vi "Open.vi"(8 "error in (no error)":errorcluster, 11 "Enabled Frames":T2={"Color"=TRUE, "Infrared"=TRUE, "LongExposureInfrared"=TRUE, "Depth"=TRUE, "BodyIndex"=TRUE, "Body"=TRUE}) -> (0 "error out":errorcluster, 3 "KinectSensor References out":T1)   [LabVIEW 2014, in "LVH-KinectOne.lvlib"]
uses:
  LVH-KinectOne.lvlib
  Private/Type Defs/KinectSensor References.ctl
  Microsoft.Kinect
  C:/github/labviewhacker/LVH-KinectOne/LabVIEW/vi.lib/LabVIEW Hacker/KinectOne/Private/Libs/BodyFrameDataInterface.dll
  Private/Libs/BodyFrameDataInterface.dll
  Private/Type Defs/FrameDescription.ctl
  Private/Frame Description FGV [Color].vi
  Private/Frame Data FGV [Color].vi
  Private/Frame Description FGV [Infrared].vi
  Private/Frame Data FGV [Infrared].vi
  Private/Frame Description FGV [Long Exposure Infrared].vi
  Private/Frame Data FGV [Long Exposure Infrared].vi
  Private/Frame Description FGV [Depth].vi
  Private/Frame Data FGV [Depth].vi
  Private/Frame Description FGV [Body Index].vi
  Private/Frame Data FGV [Body Index].vi
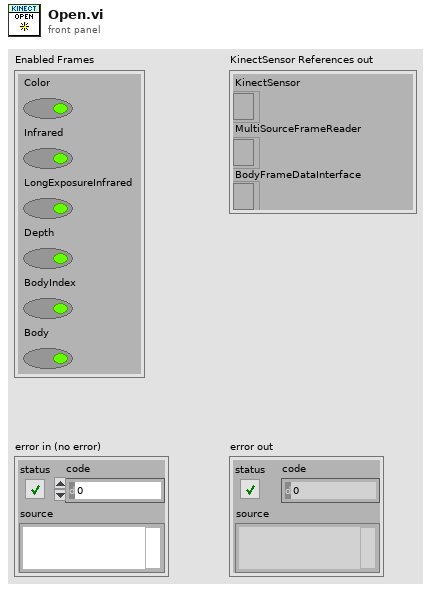
[diagram p1: front panel]
types:
  T1 = typedef "LVH-KinectOne.lvlib/KinectSensor References.ctl" = cluster{"KinectSensor":refnum<k24>, "MultiSourceFrameReader":refnum<k24>, "BodyFrameDataInterface":refnum<k24>}
  T2 = cluster{"Color":bool, "Infrared":bool, "LongExposureInfrared":bool, "Depth":bool, "BodyIndex":bool, "Body":bool}
  T3 = typedef "LVH-KinectOne.lvlib/FrameDescription.ctl" = cluster{"BytesPerPixel":u32, "DiagonalFieldOfView":sgl, "Height":i32, "HorizontalFieldOfView":sgl, "LengthInPixels":u32, "VerticalFieldOfView":sgl, "Width":i32}
  T4 = enum16{"Get Joint Position", "Initialize", "Set Joint Position"}
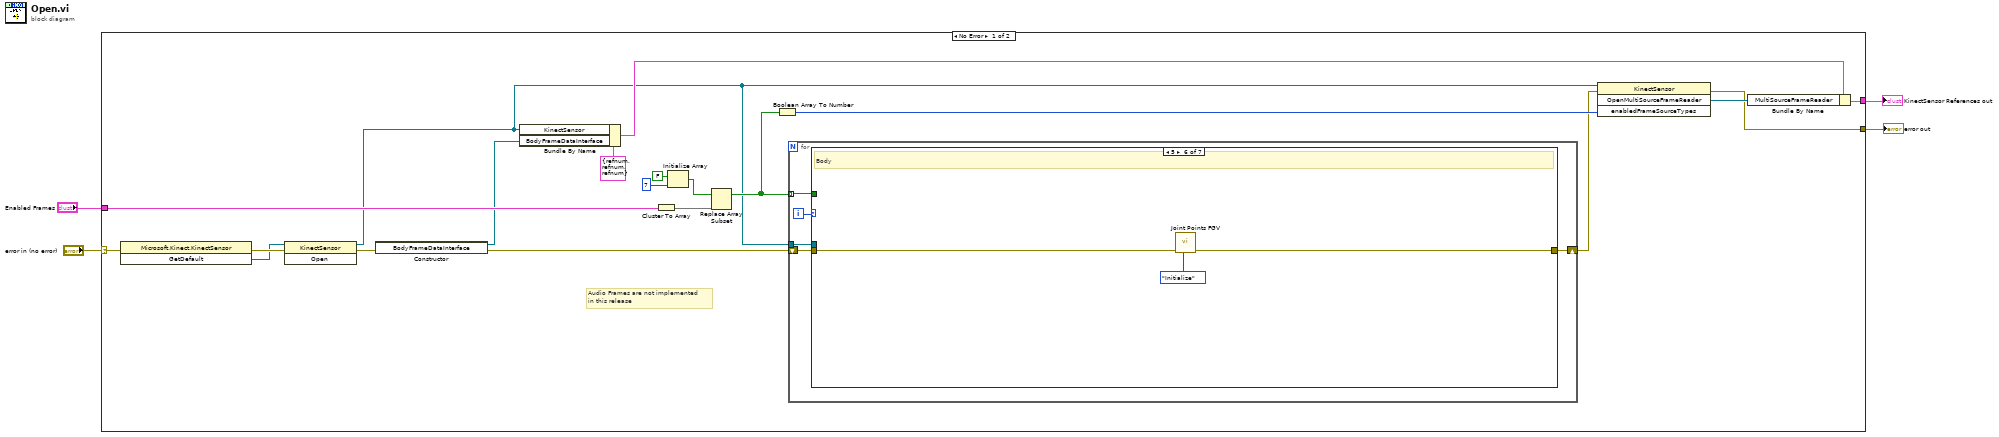
[diagram p0: block diagram]
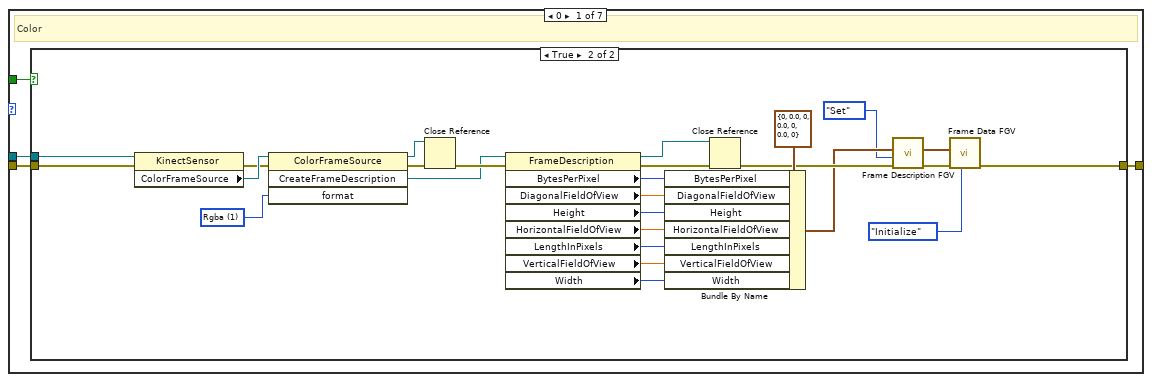
[diagram p2: hidden frame]
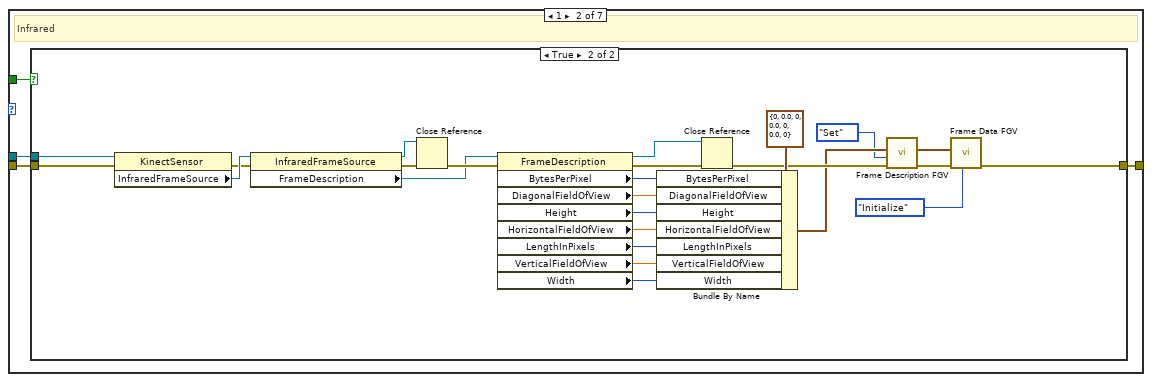
[diagram p4: hidden frame]
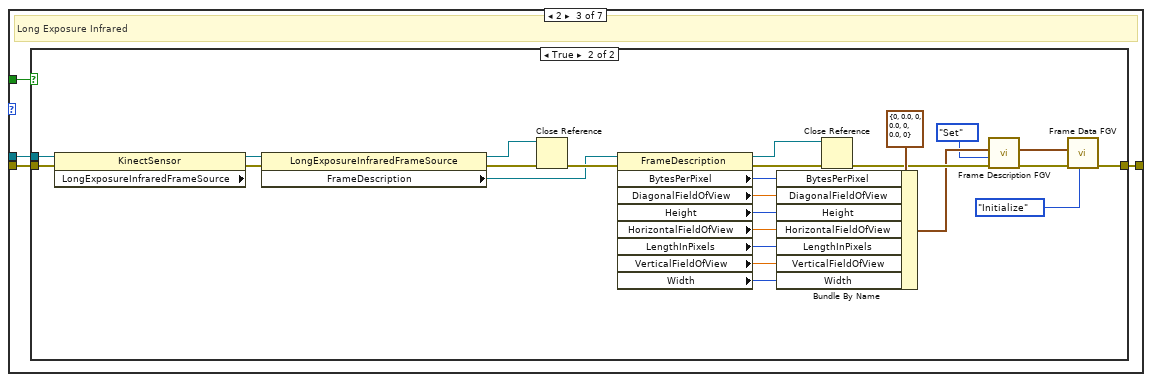
[diagram p6: hidden frame]
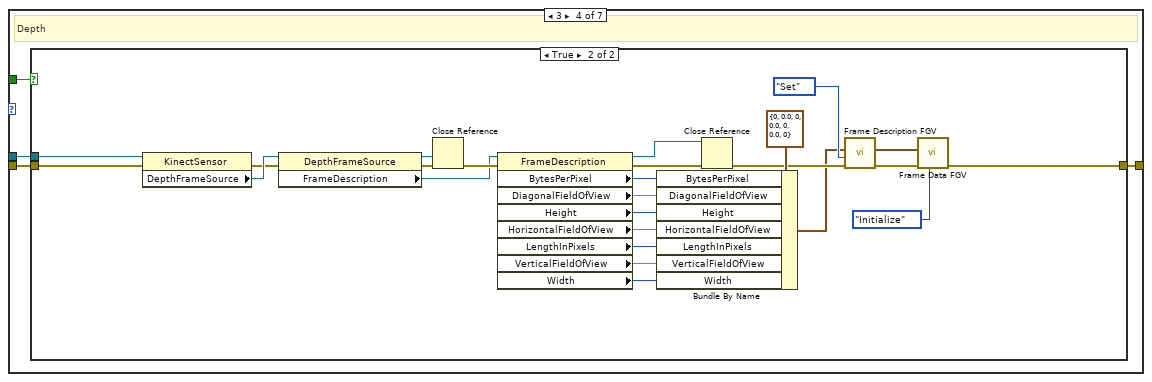
[diagram p8: hidden frame]
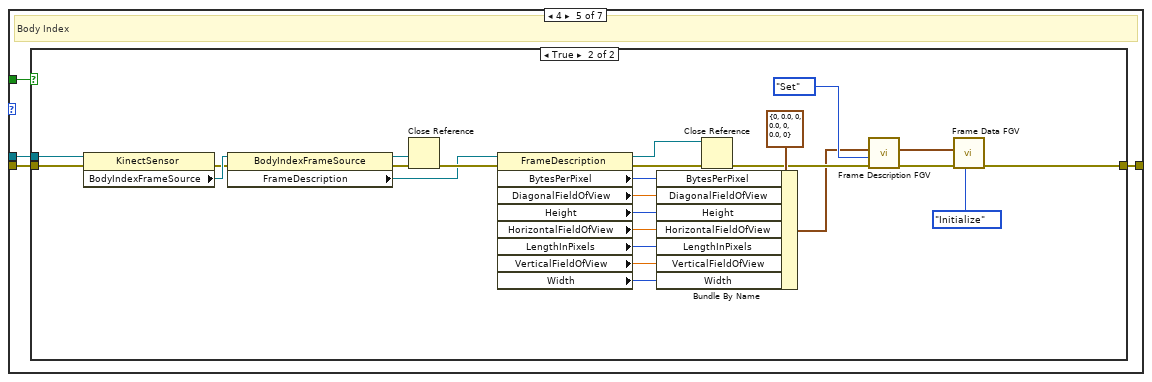
[diagram p10: hidden frame]
diagram:
  n1 = case shown="No Error" "error in (no error)" {
    selector: "error in (no error)" -> [w10 w185]
    tunnel: [w23 _] -> w4
    tunnel: "Enabled Frames" -> [w20 _]
    tunnel: [w5 w185] -> w2
    frame No Error {
      # "Audio Frames are not implemented\nin this release"
      n2 = invoke on="Invoke Node" class="Microsoft.Kinect.KinectSensor" method="GetDefault"(error in=w10) -> (error out=w13:errorcluster, "GetDefault"=w12:refnum<k24>)  [unwired: 2 in, 1 out]
      n3 = invoke class="KinectSensor" method="Open"(reference=w12, error in=w13) -> (reference out=w6:refnum<k24>, error out=w11:errorcluster)  [unwired: 1 in, 1 out]
      n4 = constructor class="BodyFrameDataInterface"(error in=w11) -> (reference out=w7:refnum<k24>, error out=w9:errorcluster)  [unwired: 2 in, 1 out]
      n5 = Bundle By Name(cluster=T1 {"KinectSensor"=refnum, "MultiSourceFrameReader"=refnum, "BodyFrameDataInterface"=refnum} ("KinectSensor References"), "KinectSensor"=w6, "BodyFrameDataInterface"=w7) -> (w8:T1)
      n6 = Cluster To Array(cluster=w20) -> (array=w16:bool[])
      n7 = Initialize Array(FALSE, 7 ("dimension size")) -> (w17:bool[])
      n8 = Replace Array Subset(array=w17, new element=w16) -> (w15:bool[])  [unwired: 1 in]
      n9 = Boolean Array To Number(Boolean array=w15) -> (number=w22:u32)
      n10 = for {
        tunnel: w15 -> [w28] mode=indexing
        shift-right: [w26] -> w21
        shift-left: w9 -> [w27]
        tunnel: w6 -> [w25]
        i -> [w29]
        n11 = case shown="5" w29 {
          tunnel: w28 -> [w33 w64 w94 w124 w154 _ _]
          tunnel: w27 -> [w32 w63 w93 w123 w153 w183 w184]
          tunnel: [w31 w62 w92 w122 w152 w182 w184] -> w26
          tunnel: w25 -> [w30 w61 w91 w121 w151 _ _]
          frame 0 {
            # "Color"
            n12 = case shown="True" w33 {
              tunnel: w32 -> [w34 w52]
              tunnel: [w34 w39] -> w31
              tunnel: w30 -> [_ w48]
              frame False {
              }
              frame True {
                w42 = 1 items=["None", "Rgba", "Yuv", "Bgra", "Bayer", "Yuy2"] ("format")
                n13 = property class="KinectSensor"(reference=w48, error in=w52) -> (error out=w43:errorcluster, "ColorFrameSource"=w46:refnum<k24>)  [unwired: 1 out]
                n14 = invoke class="ColorFrameSource" method="CreateFrameDescription"(reference=w46, error in=w43, "format"=w42) -> (reference out=w44:refnum<k24>, error out=w47:errorcluster, "CreateFrameDescription"=w45:refnum<k24>)  [unwired: 1 in, 1 out]
                n15 = Close Reference(reference=w44, error in (no error)=w47) -> (error out=w49:errorcluster)
                n16 = property class="FrameDescription"(reference=w45, error in=w49) -> (reference out=w50:refnum<k24>, error out=w51:errorcluster, "BytesPerPixel"=w54:u32, "DiagonalFieldOfView"=w55:sgl, "Height"=w56:i32, "HorizontalFieldOfView"=w57:sgl, "LengthInPixels"=w58:u32, "VerticalFieldOfView"=w59:sgl, "Width"=w60:i32)
                n17 = Bundle By Name(cluster=T3 {"BytesPerPixel"=0, "DiagonalFieldOfView"=0.0, "Height"=0, "HorizontalFieldOfView"=0.0, "LengthInPixels"=0, "VerticalFieldOfView"=0.0, "Width"=0} ("FrameDescription"), "BytesPerPixel"=w54, "DiagonalFieldOfView"=w55, "Height"=w56, "HorizontalFieldOfView"=w57, "LengthInPixels"=w58, "VerticalFieldOfView"=w59, "Width"=w60) -> (w40:T3)
                n18 = Close Reference(reference=w50, error in (no error)=w51) -> (error out=w41:errorcluster)
                n19 = call-poly "Frame Description FGV.vi"("error in (no error)"=w41, "Command"=enum16{"Get", "Set"}."Set", "FrameDescription"=w40) -> ("error out"=w38:errorcluster, "FrameDescription"=w37:T3)  [unwired: 7 in]
                n20 = call-poly "Frame Data FGV.vi"("Command"=enum16{"Get", "Initialize"}."Initialize", "error in (no error)"=w38, "FrameDescription"=w37) -> ("error out"=w39:errorcluster)  [unwired: 7 in, 1 out]
              }
            }
          }
          frame 1 {
            # "Infrared"
            n21 = case shown="True" w64 {
              tunnel: w63 -> [w65 w82]
              tunnel: [w65 w66] -> w62
              tunnel: w61 -> [_ w78]
              frame False {
              }
              frame True {
                n22 = property class="KinectSensor"(reference=w78, error in=w82) -> (error out=w76:errorcluster, "InfraredFrameSource"=w77:refnum<k24>)  [unwired: 1 out]
                n23 = property class="InfraredFrameSource"(reference=w77, error in=w76) -> (reference out=w74:refnum<k24>, error out=w75:errorcluster, "FrameDescription"=w73:refnum<k24>)
                n24 = Close Reference(reference=w74, error in (no error)=w75) -> (error out=w79:errorcluster)
                n25 = property class="FrameDescription"(reference=w73, error in=w79) -> (reference out=w80:refnum<k24>, error out=w81:errorcluster, "BytesPerPixel"=w84:u32, "DiagonalFieldOfView"=w85:sgl, "Height"=w86:i32, "HorizontalFieldOfView"=w87:sgl, "LengthInPixels"=w88:u32, "VerticalFieldOfView"=w89:sgl, "Width"=w90:i32)
                n26 = Bundle By Name(cluster=T3 {"BytesPerPixel"=0, "DiagonalFieldOfView"=0.0, "Height"=0, "HorizontalFieldOfView"=0.0, "LengthInPixels"=0, "VerticalFieldOfView"=0.0, "Width"=0} ("FrameDescription"), "BytesPerPixel"=w84, "DiagonalFieldOfView"=w85, "Height"=w86, "HorizontalFieldOfView"=w87, "LengthInPixels"=w88, "VerticalFieldOfView"=w89, "Width"=w90) -> (w71:T3)
                n27 = Close Reference(reference=w80, error in (no error)=w81) -> (error out=w72:errorcluster)
                n28 = call-poly "Frame Description FGV.vi"("error in (no error)"=w72, "Command"=enum16{"Get", "Set"}."Set", "FrameDescription"=w71) -> ("error out"=w67:errorcluster, "FrameDescription"=w68:T3)  [unwired: 7 in]
                n29 = call-poly "Frame Data FGV.vi"("Command"=enum16{"Get", "Initialize"}."Initialize", "error in (no error)"=w67, "FrameDescription"=w68) -> ("error out"=w66:errorcluster)  [unwired: 7 in, 1 out]
              }
            }
          }
          frame 2 {
            # "Long Exposure Infrared"
            n30 = case shown="True" w94 {
              tunnel: w93 -> [w95 w112]
              tunnel: [w95 w96] -> w92
              tunnel: w91 -> [_ w108]
              frame False {
              }
              frame True {
                n31 = property class="KinectSensor"(reference=w108, error in=w112) -> (error out=w106:errorcluster, "LongExposureInfraredFrameSource"=w107:refnum<k24>)  [unwired: 1 out]
                n32 = property class="LongExposureInfraredFrameSource"(reference=w107, error in=w106) -> (reference out=w104:refnum<k24>, error out=w105:errorcluster, "FrameDescription"=w103:refnum<k24>)
                n33 = Close Reference(reference=w104, error in (no error)=w105) -> (error out=w109:errorcluster)
                n34 = property class="FrameDescription"(reference=w103, error in=w109) -> (reference out=w110:refnum<k24>, error out=w111:errorcluster, "BytesPerPixel"=w114:u32, "DiagonalFieldOfView"=w115:sgl, "Height"=w116:i32, "HorizontalFieldOfView"=w117:sgl, "LengthInPixels"=w118:u32, "VerticalFieldOfView"=w119:sgl, "Width"=w120:i32)
                n35 = Bundle By Name(cluster=T3 {"BytesPerPixel"=0, "DiagonalFieldOfView"=0.0, "Height"=0, "HorizontalFieldOfView"=0.0, "LengthInPixels"=0, "VerticalFieldOfView"=0.0, "Width"=0} ("FrameDescription"), "BytesPerPixel"=w114, "DiagonalFieldOfView"=w115, "Height"=w116, "HorizontalFieldOfView"=w117, "LengthInPixels"=w118, "VerticalFieldOfView"=w119, "Width"=w120) -> (w101:T3)
                n36 = Close Reference(reference=w110, error in (no error)=w111) -> (error out=w102:errorcluster)
                n37 = call-poly "Frame Description FGV.vi"("error in (no error)"=w102, "Command"=enum16{"Get", "Set"}."Set", "FrameDescription"=w101) -> ("error out"=w97:errorcluster, "FrameDescription"=w98:T3)  [unwired: 7 in]
                n38 = call-poly "Frame Data FGV.vi"("Command"=enum16{"Get", "Initialize"}."Initialize", "error in (no error)"=w97, "FrameDescription"=w98) -> ("error out"=w96:errorcluster)  [unwired: 7 in, 1 out]
              }
            }
          }
          frame 3 {
            # "Depth"
            n39 = case shown="True" w124 {
              tunnel: w123 -> [w125 w142]
              tunnel: [w125 w131] -> w122
              tunnel: w121 -> [_ w138]
              frame False {
              }
              frame True {
                n40 = property class="KinectSensor"(reference=w138, error in=w142) -> (error out=w136:errorcluster, "DepthFrameSource"=w137:refnum<k24>)  [unwired: 1 out]
                n41 = property class="DepthFrameSource"(reference=w137, error in=w136) -> (reference out=w134:refnum<k24>, error out=w135:errorcluster, "FrameDescription"=w133:refnum<k24>)
                n42 = Close Reference(reference=w134, error in (no error)=w135) -> (error out=w139:errorcluster)
                n43 = property class="FrameDescription"(reference=w133, error in=w139) -> (reference out=w140:refnum<k24>, error out=w141:errorcluster, "BytesPerPixel"=w144:u32, "DiagonalFieldOfView"=w145:sgl, "Height"=w146:i32, "HorizontalFieldOfView"=w147:sgl, "LengthInPixels"=w148:u32, "VerticalFieldOfView"=w149:sgl, "Width"=w150:i32)
                n44 = Bundle By Name(cluster=T3 {"BytesPerPixel"=0, "DiagonalFieldOfView"=0.0, "Height"=0, "HorizontalFieldOfView"=0.0, "LengthInPixels"=0, "VerticalFieldOfView"=0.0, "Width"=0} ("FrameDescription"), "BytesPerPixel"=w144, "DiagonalFieldOfView"=w145, "Height"=w146, "HorizontalFieldOfView"=w147, "LengthInPixels"=w148, "VerticalFieldOfView"=w149, "Width"=w150) -> (w129:T3)
                n45 = Close Reference(reference=w140, error in (no error)=w141) -> (error out=w132:errorcluster)
                n46 = call-poly "Frame Description FGV.vi"("error in (no error)"=w132, "Command"=enum16{"Get", "Set"}."Set", "FrameDescription"=w129) -> ("error out"=w127:errorcluster, "FrameDescription"=w128:T3)  [unwired: 7 in]
                n47 = call-poly "Frame Data FGV.vi"("Command"=enum16{"Get", "Initialize"}."Initialize", "error in (no error)"=w127, "FrameDescription"=w128) -> ("error out"=w131:errorcluster)  [unwired: 7 in, 1 out]
              }
            }
          }
          frame 4 {
            # "Body Index"
            n48 = case shown="True" w154 {
              tunnel: w153 -> [w155 w172]
              tunnel: [w155 w161] -> w152
              tunnel: w151 -> [_ w168]
              frame False {
              }
              frame True {
                n49 = property class="KinectSensor"(reference=w168, error in=w172) -> (error out=w166:errorcluster, "BodyIndexFrameSource"=w167:refnum<k24>)  [unwired: 1 out]
                n50 = property class="BodyIndexFrameSource"(reference=w167, error in=w166) -> (reference out=w164:refnum<k24>, error out=w165:errorcluster, "FrameDescription"=w163:refnum<k24>)
                n51 = Close Reference(reference=w164, error in (no error)=w165) -> (error out=w169:errorcluster)
                n52 = property class="FrameDescription"(reference=w163, error in=w169) -> (reference out=w170:refnum<k24>, error out=w171:errorcluster, "BytesPerPixel"=w174:u32, "DiagonalFieldOfView"=w175:sgl, "Height"=w176:i32, "HorizontalFieldOfView"=w177:sgl, "LengthInPixels"=w178:u32, "VerticalFieldOfView"=w179:sgl, "Width"=w180:i32)
                n53 = Bundle By Name(cluster=T3 {"BytesPerPixel"=0, "DiagonalFieldOfView"=0.0, "Height"=0, "HorizontalFieldOfView"=0.0, "LengthInPixels"=0, "VerticalFieldOfView"=0.0, "Width"=0} ("FrameDescription"), "BytesPerPixel"=w174, "DiagonalFieldOfView"=w175, "Height"=w176, "HorizontalFieldOfView"=w177, "LengthInPixels"=w178, "VerticalFieldOfView"=w179, "Width"=w180) -> (w159:T3)
                n54 = Close Reference(reference=w170, error in (no error)=w171) -> (error out=w162:errorcluster)
                n55 = call-poly "Frame Description FGV.vi"("error in (no error)"=w162, "Command"=enum16{"Get", "Set"}."Set", "FrameDescription"=w159) -> ("error out"=w157:errorcluster, "FrameDescription"=w158:T3)  [unwired: 7 in]
                n56 = call-poly "Frame Data FGV.vi"("Command"=enum16{"Get", "Initialize"}."Initialize", "error in (no error)"=w157, "FrameDescription"=w158) -> ("error out"=w161:errorcluster)  [unwired: 7 in, 1 out]
              }
            }
          }
          frame 5 {
            # "Body"
            n57 = call "Joint Points FGV.vi"("Command"=T4."Initialize", "error in (no error)"=w183) -> ("error out"=w182:errorcluster)  [unwired: 8 in, 1 out]
          }
          frame 6, Default {
            # "Default"
          }
        }
      }
      n58 = invoke class="KinectSensor" method="OpenMultiSourceFrameReader"(reference=w6, error in=w21, "enabledFrameSourceTypes"=w22) -> (error out=w5:errorcluster, "OpenMultiSourceFrameReader"=w24:refnum<k24>)  [unwired: 1 in, 2 out]
      n59 = Bundle By Name(cluster=w8, "MultiSourceFrameReader"=w24) -> (w23:T1)
    }
    frame Error {
      # "Pass out upstream error"
    }
  }
  "error out" <- w2
  "KinectSensor References out" <- w4
